vi "Set Cycles AI Filter.vi"(0 "FPGA API in":refnum<class "FPGA API.lvclass">, 5 "Cycles to Filter":u16, 11 "error in (no error)":errorcluster) -> (4 "FPGA API out":refnum<class "FPGA API.lvclass">, 15 "error out":errorcluster)   [LabVIEW 2019, in "FPGA API.lvclass"]
uses:
  FPGA API.lvclass
  FPGA API.lvclass/FPGA API.ctl
  <vilib>/Utility/error.llb/Error Cluster From Error Code.vi
  <vilib>/rvi/errors/niLvFpgaAdjustHostInterfaceError.vi
  <vilib>/rvi/interface/nirviReadWriteControl/nirviReadWriteControl.xnode
  FPGA Ref.ctl
  NiFpgaLv.dll
  <vilib>/rvi/interface/Simulation/niFpgaSimulationCallBeginRW.vi
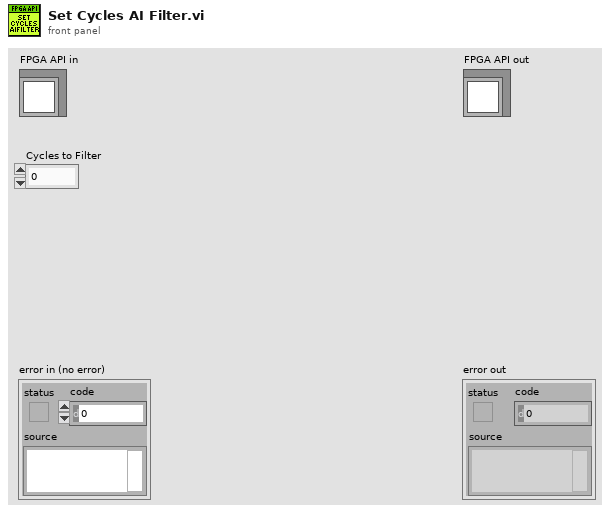
[diagram p1: front panel]
types:
  T1 = typedef "FPGA API.lvclass/FPGA Ref.ctl" = refnum<k20>
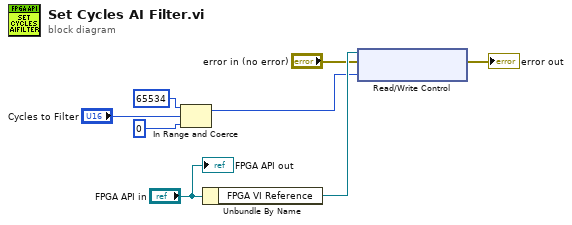
[diagram p0: block diagram]
diagram:
  n1 = In Range and Coerce(upper limit=u16 65534, x="Cycles to Filter", lower limit=u16 0) -> (coerced(x)=w4:u16)  [unwired: 1 out]
  n2 = Unbundle By Name("FPGA API in") -> ("FPGA VI Reference"=w7:T1)
  n3 = xnode "Read/Write Control"("FPGA VI Reference In"=w7, "error in"="error in (no error)", "Cycles to Filter AI"=w4) -> ("error out"=→"error out":errorcluster)  [unwired: 1 out]
  "FPGA API out" <- "FPGA API in"
